vi "Format Client Request (Numeric).vi"(8 "error in (no error)":errorcluster, 9 "id":i32, 10 "params":variant, 11 "method":string) -> (0 "error out":errorcluster, 2 "Request String":string)   [LabVIEW 2015, in "JSONRPC Server.lvclass"]
uses:
  JSONRPC Server.lvclass
  <vilib>/NI/i3 JSON/JSON Generation/Add Object Parameter Files/Add Object Parameter - Numeric.vi
  <vilib>/NI/i3 JSON/i3-json.lvlib
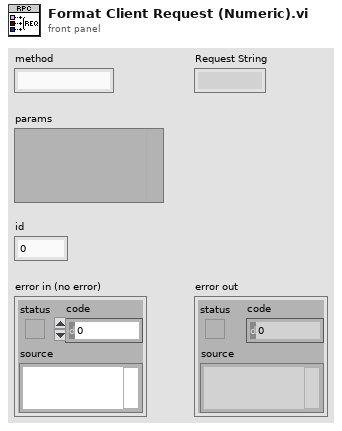
[diagram p1: front panel]
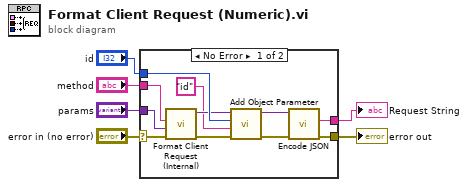
[diagram p0: block diagram]
diagram:
  n1 = case shown="No Error" "error in (no error)" {
    selector: "error in (no error)" -> [w17 w18]
    tunnel: [w16 w18] -> w5
    tunnel: "params" -> [w7 _]
    tunnel: [w15 _] -> w3
    tunnel: "method" -> [w14 _]
    tunnel: "id" -> [w13 _]
    frame No Error {
      n2 = call "Format Client Request (Internal).vi"("error in (no error)"=w17, "params"=w7, "method"=w14) -> ("error out"=w9:errorcluster, "JSON Tree out (JSON Object)"=w12:variant)  [unwired: 7 in]
      n3 = call-poly <vilib>:"Add Object Parameter.vi"("error in (no error)"=w9, "Name"="id", "Numeric"=w13, "JSON Tree in (JSON Object)"=w12) -> ("error out"=w10:errorcluster, "JSON Tree out (JSON Object)"=w11:variant)  [unwired: 6 in]
      n4 = call <vilib>:"Encode JSON.vi"("error in (no error)"=w10, "JSON Tree In"=w11) -> ("error out"=w16:errorcluster, "String"=w15:string)  [unwired: 4 in]
    }
    frame Error {
    }
  }
  "error out" <- w5
  "Request String" <- w3
